vi "读取固件状态.vi"(8 "错误输入":errorcluster, 11 "MB session in":refnum<class "MB_Master.lvclass">) -> (0 "error out":errorcluster, 2 "结果字符串":string, 3 "MB session out":refnum<class "MB_Master.lvclass">)   [LabVIEW 2016, in "斯坦道总磷.lvlib"]
uses:
  <vilib>/Plasmionique/MB Master/MB_Master/MB_Master.lvclass
  <vilib>/Plasmionique/MB Master/MB_Master_Serial/MB_Master_Serial.lvclass
  C:/Program Files (x86)/National Instruments/LabVIEW 2016/vi.lib/Plasmionique/MB Master/MB_Master/MB_Master.lvclass
  <vilib>/Plasmionique/MB Master/MB Master.lvlib
panel:
  in  "VISA Resource":refnum<visa-resource-name>
  in  "引用选择":enum16{"MB引用", "自建引用"}(ring)
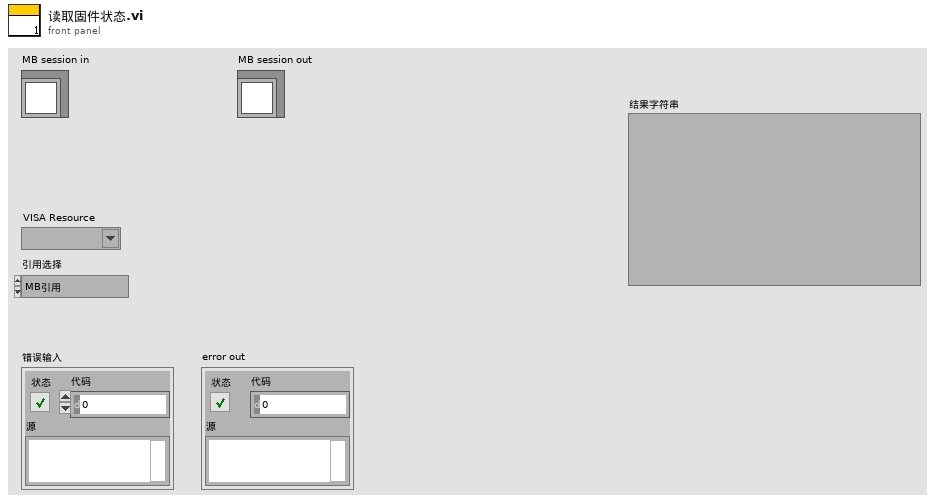
[diagram p1: front panel]
types:
  T1 = cluster{"baud rate (bps)":u32, "stop bits":u16, "parity":u16, "flow control":u16, "timeout":u32, "retries":i32}
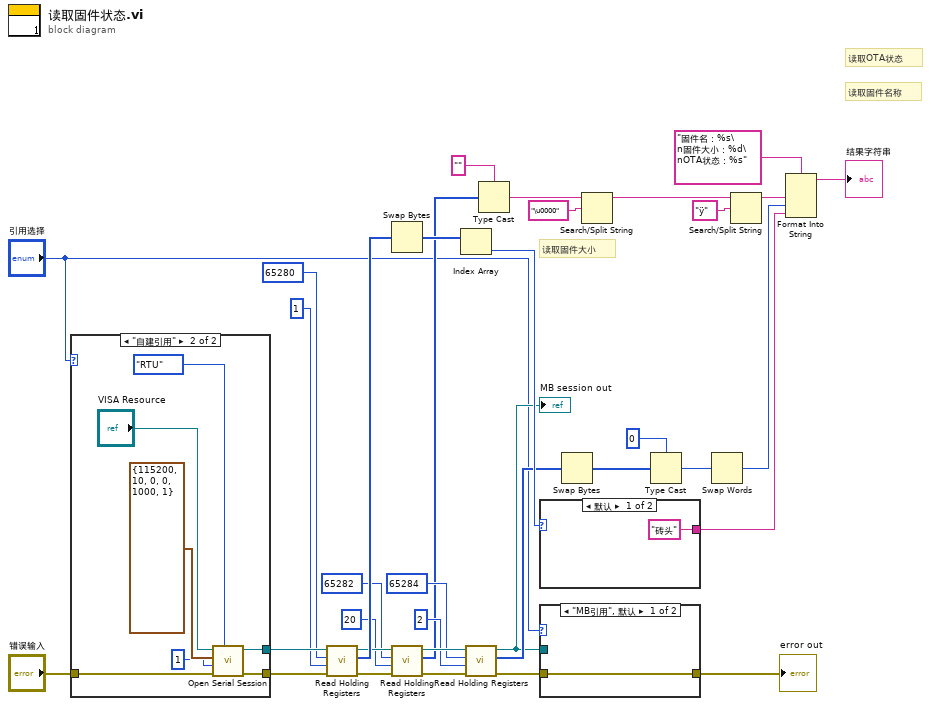
[diagram p0: block diagram]
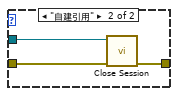
[diagram p2: hidden frame]
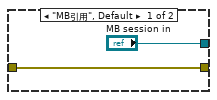
[diagram p3: hidden frame]
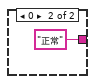
[diagram p4: hidden frame]
diagram:
  # "读取固件大小"
  # "读取固件名称"
  # "读取OTA状态"
  n1 = case shown="\"自建引用\"" "引用选择" {
    tunnel: ["MB session in" w43] -> w34
    tunnel: "错误输入" -> [w36 w42]
    tunnel: [w36 w41] -> w13
    frame "MB引用", Default {
    }
    frame "自建引用" {
      n2 = call <vilib>:"Open Serial Session.vi"("Mode (RTU)"=enum16{"RTU", "ASCII"}."RTU", "Error in"=w42, "Slave ID"=u8 1, "Serial Config"=T1 {"baud rate (bps)"=115200, "stop bits"=10, "parity"=0, "flow control"=0, "timeout"=1000, "retries"=1}, "VISA Resource"="VISA Resource") -> ("Error out"=w41:errorcluster, "MB_Serial session"=w43:refnum<class "MB_Master_Serial.lvclass">)  [unwired: 5 in]
    }
  }
  n3 = call <vilib>:"Read Holding Registers.vi"("error in (no error)"=w13, "quantity"=u16 1, "starting address"=u16 65280, "MB session in"=w34) -> ("error out"=w21:errorcluster, "Registers"=w31:u16[], "MB session out"=w26:refnum<class "MB_Master.lvclass">)  [unwired: 5 in]
  n4 = Swap Bytes(anything=w31) -> (byte swapped=w29:u16[])
  n5 = call <vilib>:"Read Holding Registers.vi"("error in (no error)"=w21, "quantity"=u16 20, "starting address"=u16 65282, "MB session in"=w26) -> ("error out"=w20:errorcluster, "Registers"=w8:u16[], "MB session out"=w24:refnum<class "MB_Master.lvclass">)  [unwired: 5 in]
  n6 = Index Array(array=w29) -> (element=w30:u16)  [unwired: 1 in]
  n7 = call <vilib>:"Read Holding Registers.vi"("error in (no error)"=w20, "quantity"=u16 2, "starting address"=u16 65284, "MB session in"=w24) -> ("error out"=w6:errorcluster, "Registers"=w19:u16[], "MB session out"=w7:refnum<class "MB_Master.lvclass">)  [unwired: 5 in]
  "MB session out" <- w7
  n8 = Type Cast(type="", x=w8) -> (*(type *) &x=w9:string)
  n9 = case shown="默认" w30 {
    tunnel: ["砖头" "正常"] -> w28
    frame Default {
    }
    frame 0 {
    }
  }
  n10 = case shown="\"MB引用\", 默认" "引用选择" {
    tunnel: w7 -> [_ w50]
    tunnel: w6 -> [w47 w49]
    tunnel: [w47 w48] -> w5
    frame "MB引用", Default {
    }
    frame "自建引用" {
      n11 = call-dynamic "Close Session.vi"("error in (no error)"=w49, "MB session in"=w50) -> ("error out"=w48:errorcluster)  [unwired: 9 in]
    }
  }
  "error out" <- w5
  n12 = Swap Bytes(anything=w19) -> (byte swapped=w18:u16[])
  n13 = Search/Split String(string=w9, search string/char (-)="\u0000" ("搜索字符串")) -> (substring before match=w3:string)  [unwired: 1 in, 2 out]
  n14 = Type Cast(type=u32 0, x=w18) -> (*(type *) &x=w16:u32)
  n15 = Swap Words(1:w16) -> (0:w15:u32)
  n16 = Search/Split String(string=w3, search string/char (-)="ÿ" ("搜索字符串")) -> (substring before match=w2:string)  [unwired: 1 in, 2 out]
  n17 = Format Into String(format string="固件名：%s\n固件大小：%d\nOTA状态：%s" ("格式字符串"), w2, w15, w28) -> (resulting string=→"结果字符串":string)  [unwired: 2 in, 1 out]
